vi "Run Command.vi"(8 "error in (no error)":errorcluster, 10 "command":T1, 11 "Thread in":refnum<class "Thread.lvclass">) -> (0 "error out":errorcluster, 1 "shutdown?":bool, 3 "Thread out":refnum<class "Thread.lvclass">)   [LabVIEW 2017, in "DSF Core.lvlib" / "Thread.lvclass"]
uses:
  Thread.lvclass
  Thread Command.ctl
  Thread State.ctl
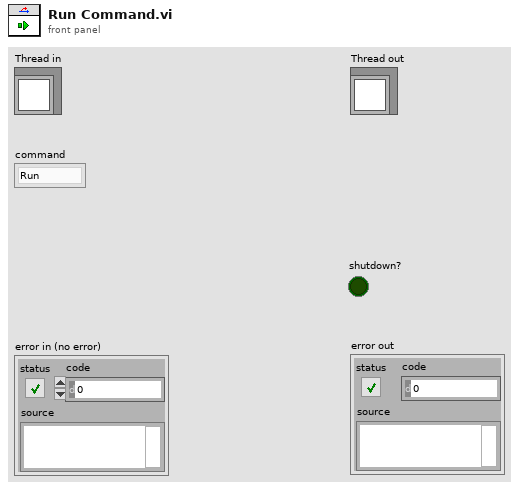
[diagram p1: front panel]
types:
  T1 = typedef "DSF Core.lvlib/Thread.lvclass/Thread Command.ctl" = enum8{"Run", "Shutdown"}
  T2 = typedef "DSF Core.lvlib/Thread.lvclass/Thread State.ctl" = enum8{"Idle", "Running", "Error", "Shut Down"}
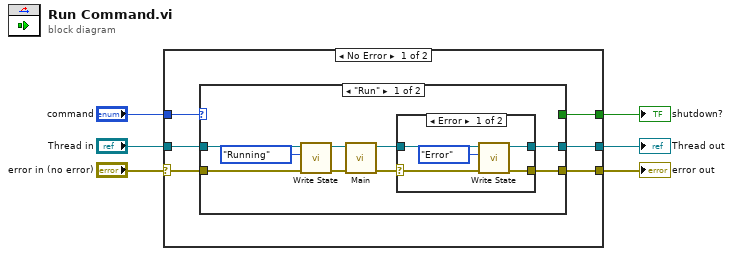
[diagram p0: block diagram]
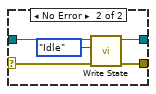
[diagram p2: hidden frame]
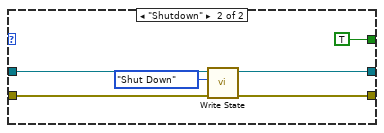
[diagram p3: hidden frame]
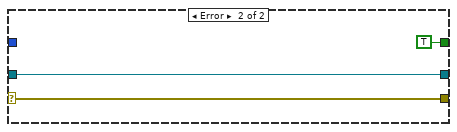
[diagram p4: hidden frame]
diagram:
  n1 = case shown="No Error" "error in (no error)" {
    selector: "error in (no error)" -> [w7 w40]
    tunnel: "command" -> [w12 _]
    tunnel: "Thread in" -> [w11 w39]
    tunnel: [w10 w39] -> w4
    tunnel: [w9 w40] -> w3
    tunnel: [w8 TRUE] -> w2
    frame No Error {
      n2 = case shown="\"Run\"" w12 {
        tunnel: w7 -> [w20 w34]
        tunnel: [w13 w32] -> w9
        tunnel: [w14 w33] -> w10
        tunnel: w11 -> [w21 w35]
        tunnel: [_ TRUE] -> w8
        frame "Run" {
          n3 = call "Write State.vi"("error in (no error)"=w20, "state"=Thread_State."Running", "Thread in"=w21) -> ("error out"=w18:errorcluster, "Thread out"=w19:refnum<class "Thread.lvclass">)  [unwired: 7 in]
          n4 = call-dynamic "Main.vi"("error in (no error)"=w18, "Thread in"=w19) -> ("error out"=w16:errorcluster, "Thread out"=w15:refnum<class "Thread.lvclass">)  [unwired: 8 in]
          n5 = case shown="Error" w16 {
            selector: w16 -> [w24 w29]
            tunnel: w15 -> [w25 w30]
            tunnel: [w23 w28] -> w14
            tunnel: [w22 w27] -> w13
            frame Error {
              n6 = call "Write State.vi"("error in (no error)"=w24, "state"=Thread_State."Error", "Thread in"=w25) -> ("error out"=w22:errorcluster, "Thread out"=w23:refnum<class "Thread.lvclass">)  [unwired: 7 in]
            }
            frame No Error {
              n7 = call "Write State.vi"("error in (no error)"=w29, "state"=Thread_State."Idle", "Thread in"=w30) -> ("error out"=w27:errorcluster, "Thread out"=w28:refnum<class "Thread.lvclass">)  [unwired: 7 in]
            }
          }
        }
        frame "Shutdown" {
          n8 = call "Write State.vi"("error in (no error)"=w34, "state"=Thread_State."Shut Down", "Thread in"=w35) -> ("error out"=w32:errorcluster, "Thread out"=w33:refnum<class "Thread.lvclass">)  [unwired: 7 in]
        }
      }
    }
    frame Error {
    }
  }
  "Thread out" <- w4
  "error out" <- w3
  "shutdown?" <- w2
